vi "Monitor Datum.vi"(8 "Time Stamp":timestamp, 9 "Datum":variant, 10 "Name":string, 11 "MediatorBusMonitor In":refnum<class "MediatorBusMonitor.lvclass">) -> (0 "error out":errorcluster, 3 "MediatorBusMonitor Out":refnum<class "MediatorBusMonitor.lvclass">)   [LabVIEW 2017, in "MyMediator.lvlib副本.lvlib" / "MediatorBusMonitor.lvclass"]
uses:
  MediatorBusMonitor/MediatorBusMonitor.lvclass
  MediatorBusMonitor/MediatorBusMonitor.lvclass/MediatorBusMonitor.ctl
  <vilib>/Composed/GPM Packages/lookup-table/Source/LookupTable/LookupTable.lvclass/LookupTable.ctl
  fcb8a66a-8ef2-493c-af54-0c2a0b210573.vi
  <vilib>/Composed/GPM Packages/lookup-table/Source/LookupTable/Read Table Reference.vi
  fcb8a66a-8ef2-493c-af54-0c2a0b210573.vi/60d731ab-cc56-440f-aed9-426a382ef668.vi
  <vilib>/Composed/GPM Packages/lookup-table/Source/LookupTable/LookupTable.lvclass
  <vilib>/Composed/GPM Packages/variant/Source/VariantExtensions.lvlib
panel:
  in  "error in (no error)":errorcluster
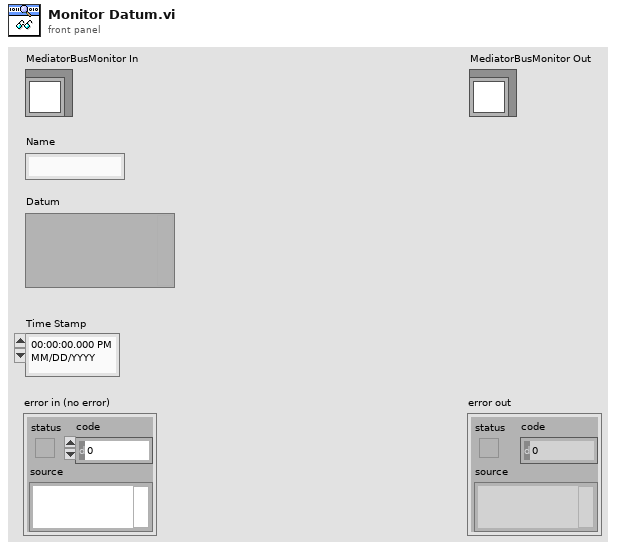
[diagram p1: front panel]
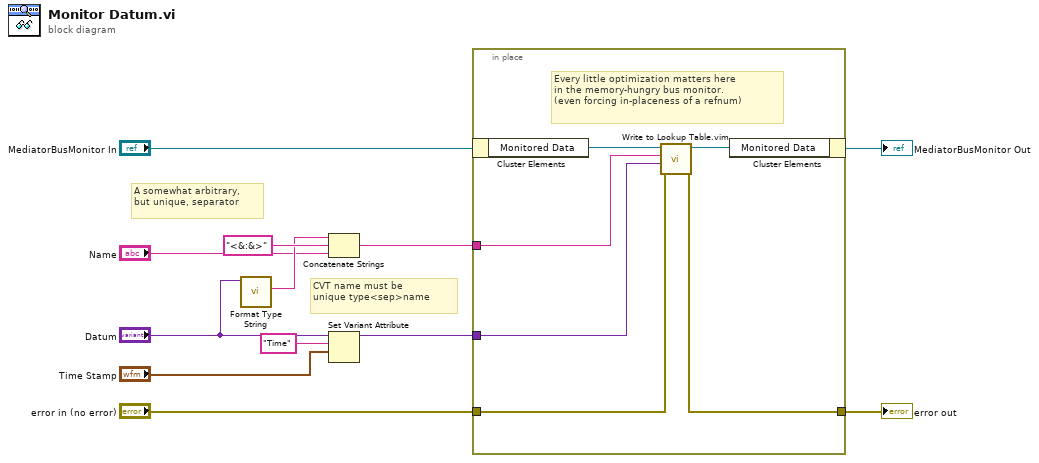
[diagram p0: block diagram]
diagram:
  # "A somewhat arbitrary,\nbut unique, separator"
  # "CVT name must be\nunique type<sep>name"
  n1 = call <vilib>:"Format Type String.vi"("Data Type"="Datum") -> ("Type Name"=w9:string)  [unwired: 9 in, 1 out]
  n2 = Concatenate Strings(w9, "<&:&>" ("string"), "Name") -> (w8:string)
  n3 = Set Variant Attribute(Variant="Datum", name="Time", value="Time Stamp") -> (Variant out=w11:variant)  [unwired: 1 in, 2 out]
  n4 = in-place {
    in-place-border: w11 -> [w18]
    in-place-border: w8 -> [w17]
    in-place-border: "error in (no error)" -> [w14]
    in-place-border: [w13] -> w1
    # "Every little optimization matters here\nin the memory-hungry bus monitor.\n(even forcing in-placeness of a refnum)"
    n5 = in-place-cluster #1("MediatorBusMonitor In") -> ("Monitored Data"=w16:refnum<data-value>)
    n6 = call "Write to Lookup Table.vim"("error in (no error)"=w14, "Item"=w18, "Item Name"=w17, "LookupTable Reference"=w16) -> ("error out"=w13:errorcluster, "LookupTable Reference Out"=w15:refnum<data-value>)  [unwired: 5 in, 1 out]
    n7 = in-place-cluster #1("Monitored Data"=w15) -> (→"MediatorBusMonitor Out":refnum<class "MediatorBusMonitor.lvclass">)
  }
  "error out" <- w1
